vi "Untitled 5.vi"   [LabVIEW 2017]
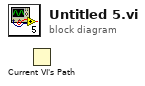
[diagram p0: block diagram]
diagram:
  n1 = Current VI's Path() -> ()  [unwired: 1 out]
